vi "Modbus Read U8.vi"(7 "Slave Address":u8, 8 "error in (no error)":errorcluster, 10 "Register Start Address":u16 format="%x", 11 "VISA resource in":refnum<visa-resource-name>) -> (0 "error out":errorcluster, 1 "Output data U8":u8, 3 "VISA resource out":refnum<visa-resource-name>)   [LabVIEW 2023, in "Voegtlin_NI_SMART_Modbus_Drivers.lvlib"]
doc: "Lese einen U8-Werte an der angegebenen Startadresse des selektierten Geraetes aus.\nDer COM-Port muss dazu initialisiert sein (benutze\" Modbus Init.vi\")."
uses:
  Voegtlin_NI_SMART_Modbus_Drivers.lvlib
  Enums/Modbus Comm.ctl
panel:
  out "Read register data\n U16 (array)":u16[](array[numeric])
  # "Input Data"
  # "Internal Data"
  # "Output Data"
  # "(Inputmaske in HEX)"
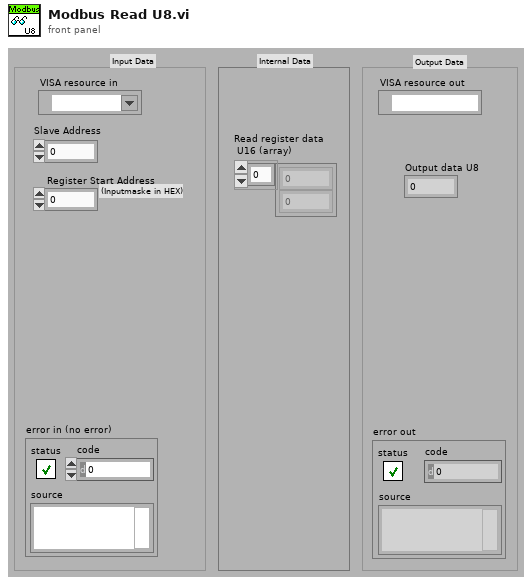
[diagram p1: front panel]
types:
  T1 = typedef "Voegtlin_NI_SMART_Modbus_Drivers.lvlib/Modbus Comm.ctl" = enum16{"Init", "Read", "Write", "Exit"}
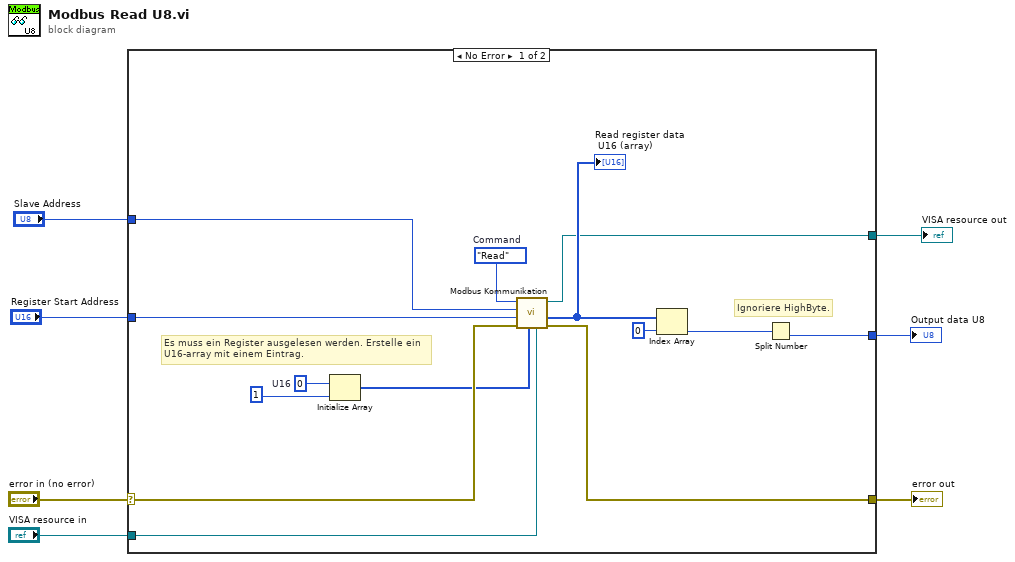
[diagram p0: block diagram]
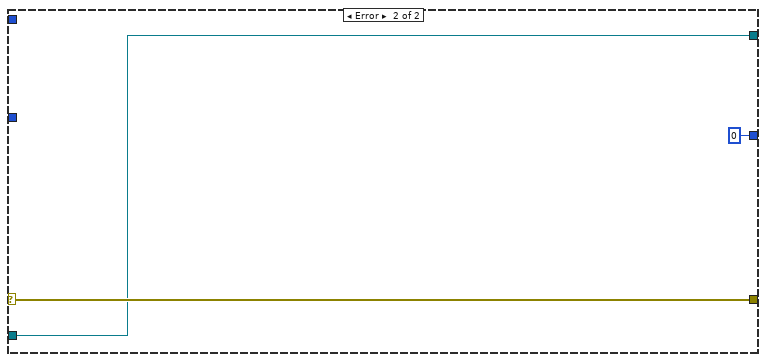
[diagram p2: hidden frame]
diagram:
  n1 = case shown="No Error" "error in (no error)" {
    selector: "error in (no error)" -> [w13 w24]
    tunnel: "Register Start Address" -> [w11 _]
    tunnel: [w21 w24] -> w6
    tunnel: [w17 u8 0] -> w5
    tunnel: "Slave Address" -> [w10 _]
    tunnel: "VISA resource in" -> [w9 w22]
    tunnel: [w8 w22] -> w1
    frame No Error {
      w19 = u16 0  # U16
      w20 = Modbus_Comm."Read"  # Command
      # "Ignoriere HighByte."
      # "Es muss ein Register ausgelesen werden. Erstelle ein U16-array mit einem Eintrag."
      n2 = Initialize Array(w19, u16 1 ("Number of U8 to read")) -> (w12:u16[])
      n3 = call "Modbus Kommunikation.vi"("VISA resource in"=w9, "Data In / #Reads [U16]"=w12, "error in (no error)"=w13, "Register Start Address"=w11, "Slave Address"=w10, "Command"=w20) -> ("error out"=w21:errorcluster, "Data Out [U16]"=w14:u16[], "VISA resource out"=w8:refnum<visa-resource-name>)  [unwired: 3 in]
      "Read register data\n U16 (array)" <- w14
      n4 = Index Array(array=w14, index=u16 0 ("Number of U8 to read")) -> (element=w15:u16)
      n5 = Split Number(x=w15) -> (lo(x)=w17:u8)  [unwired: 1 out]
    }
    frame Error {
    }
  }
  "error out" <- w6
  "Output data U8" <- w5
  "VISA resource out" <- w1
